vi "Get Disable Buffering.vi"(8 "error in (no error)":errorcluster, 11 "Log File Specification in":refnum<class "Log File Specification.lvclass">) -> (0 "error out":errorcluster, 2 "Disable Buffering":bool, 3 "Log File Specification out":refnum<class "Log File Specification.lvclass">)   [LabVIEW 2015, in "Waveform Data Logger Shared.lvlib" / "Log File Specification.lvclass"]
uses:
  Log File Specification.lvclass
  Log File Specification.lvclass/Log File Specification.ctl
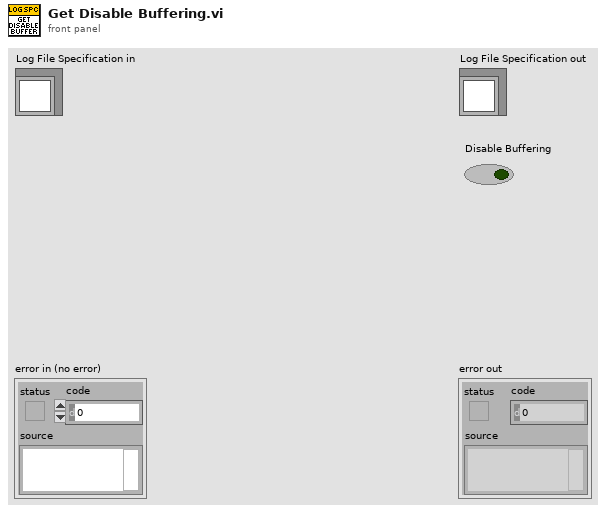
[diagram p1: front panel]
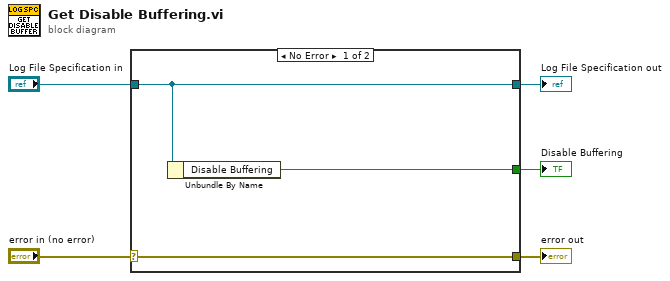
[diagram p0: block diagram]
diagram:
  n1 = case shown="No Error" "error in (no error)" {
    selector: "error in (no error)" -> [w8 w9]
    tunnel: [w8 w9] -> w4
    tunnel: [w7 w10] -> w2
    tunnel: "Log File Specification in" -> [w7 w10]
    tunnel: [w6 _] -> w1
    frame No Error {
      n2 = Unbundle By Name(w7) -> ("Disable Buffering"=w6:bool)
    }
    frame Error {
    }
  }
  "error out" <- w4
  "Log File Specification out" <- w2
  "Disable Buffering" <- w1
